vi "Setup Waveform Measurement.vi"(6 "error in (no error)":errorcluster, 8 "Function":T1, 9 "Driver":refnum<class "Driver.lvclass">) -> (0 "error out":errorcluster, 2 "Id":string, 3 "CommandDirector":refnum<class "CommandDirector.lvclass">)   [LabVIEW 2023]
uses:
  Driver/Driver.lvclass
  Measure/Measure Function.ctl
  CommandDirector/CommandDirector.lvclass
  Measure/Measure.lvclass
  \\Mac\Home/Documents/LabVIEW Data/ProjectTemplates/Source/HAF/WriteCommand/WriteCommand.lvclass
  ContinuousDirector/ContinuousDirector.lvclass
  \\Mac\Home/Documents/LabVIEW Data/ProjectTemplates/Source/HAF/CommandDirector/CommandDirector.lvclass
  Parameter/Parameter.lvclass
  HAF.lvlib
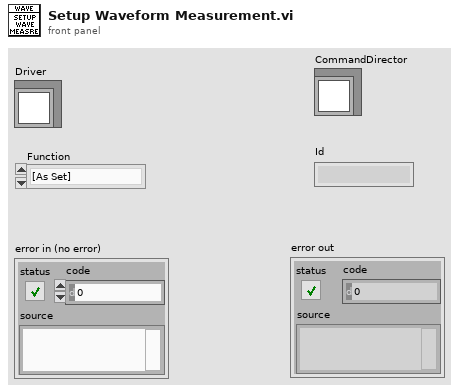
[diagram p1: front panel]
types:
  T1 = typedef "HAF.lvlib/Measure Function.ctl" = enum16{"[As Set]", "DC Voltage", "AC Voltage", "DC Current", "AC Current", "2-wire Resistance", "4-wire Resistance", "Diode", "Capacitance", "Temperature", "Continuity", "Frequency", "Period", "DC Voltage Ratio"}
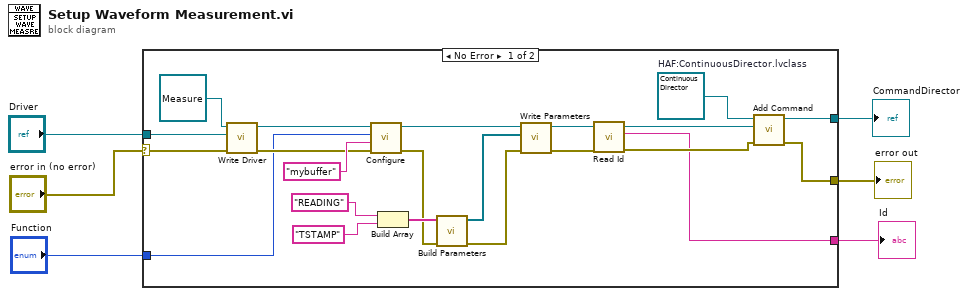
[diagram p0: block diagram]
diagram:
  n1 = case shown="No Error" "error in (no error)" {
    selector: "error in (no error)" -> [w26 w29]
    tunnel: "Driver" -> [w27 _]
    tunnel: "Function" -> [w22 _]
    tunnel: [w9 _] -> w3
    tunnel: [w8 _] -> w2
    tunnel: [w7 w29] -> w1
    frame No Error {
      w12 = refnum<class "ContinuousDirector.lvclass"> refnum  # HAF:ContinuousDirector.lvclass
      n2 = call-dynamic "Write Driver.vi"("error in (no error)"=w26, "HAF:Driver.lvclass"=w27, "WriteCommand in"=refnum<class "Measure.lvclass"> refnum ("HAF:Measure.lvclass")) -> ("error out"=w23:errorcluster, "WriteCommand out"=w25:refnum<class "Measure.lvclass">)  [unwired: 7 in]
      n3 = call-dynamic "Configure.vi"("error in (no error)"=w23, "Buffer"="mybuffer", "Function"=w22, "Measure in"=w25) -> ("error out"=w17:errorcluster, "Measure out"=w21:refnum<class "Measure.lvclass">)  [unwired: 6 in]
      n4 = Build Array("READING", "TSTAMP") -> (w18:string[])
      n5 = call "Build Parameters.vi"("error in (no error)"=w17, "Parameter Names"=w18) -> ("error out"=w15:errorcluster, "Parameters"=w16:refnum<class "Parameter.lvclass">[])  [unwired: 8 in]
      n6 = call-dynamic "Write Parameters.vi"("error in (no error)"=w15, "Parameters"=w16, "WriteCommand in"=w21) -> ("error out"=w13:errorcluster, "WriteCommand out"=w14:refnum<class "Measure.lvclass">)  [unwired: 7 in]
      n7 = call-dynamic "Read Id.vi"("error in (no error)"=w13, "WriteCommand in"=w14) -> ("error out"=w10:errorcluster, "Id"=w8:string, "WriteCommand out"=w11:refnum<class "Measure.lvclass">)  [unwired: 7 in]
      n8 = call-dynamic "Add Command.vi"("error in (no error)"=w10, "Write Command"=w11, "Command Director in"=w12) -> ("error out"=w7:errorcluster, "Command Director out"=w9:refnum<class "ContinuousDirector.lvclass">)  [unwired: 7 in]
    }
    frame Error {
    }
  }
  "error out" <- w1
  "CommandDirector" <- w3
  "Id" <- w2
